vi "SVPO Limit Testing.vi"   [LabVIEW 2017, in "SoundVib_LimitTest.lvlib"]
doc: "Performs limit testing on single-precision waveforms, single-precision scaled arrays, or double-precision scalar measurements. You can specify an upper and lower boundary of the envelope to define a pass range. This VI uses the defined pass range to test the input signal. VI outputs apply to all the tests since the last VI reset. Use this VI on embedded targets that have limited computational resources. Wire data to the <B>value in</B> input to determine the polymorphic instance to use or manually select the instance."
uses:
  <vilib>/addons/Sound and Vibration/svt_Limit Test/SoundVib_LimitTest.lvlib
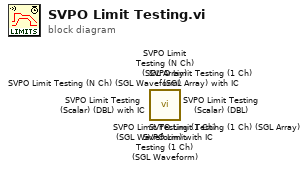
[diagram p0: block diagram]
diagram:
  n1 = call <vilib>:"SVPO Limit Testing (1 Ch) (SGL Waveform) with IC.vi"() -> ()  [unwired: 7 in, 5 out]
  n2 = call <vilib>:"SVPO Limit Testing (1 Ch) (SGL Array) with IC.vi"() -> ()  [unwired: 8 in, 4 out]
  n3 = call <vilib>:"SVPO Limit Testing (Scalar) (DBL) with IC.vi"() -> ()  [unwired: 8 in, 4 out]
  n4 = call <vilib>:"SVPO Limit Testing (Scalar) (DBL).vi"() -> ()  [unwired: 9 in, 3 out]
  n5 = call <vilib>:"SVPO Limit Testing (N Ch) (SGL Waveform).vi"() -> ()  [unwired: 8 in, 4 out]
  n6 = call <vilib>:"SVPO Limit Testing (N Ch) (SGL Array).vi"() -> ()  [unwired: 9 in, 3 out]
  n7 = call <vilib>:"SVPO Limit Testing (1 Ch) (SGL Waveform).vi"() -> ()  [unwired: 8 in, 4 out]
  n8 = call <vilib>:"SVPO Limit Testing (1 Ch) (SGL Array).vi"() -> ()  [unwired: 9 in, 3 out]
